vi "Get Unified Force.vi"(10 "diameter results":dbl[][](array[numeric]), 11 "force results":dbl[][](array[numeric])) -> (3 "unified force array":dbl[](array[numeric]))   [LabVIEW 2020]
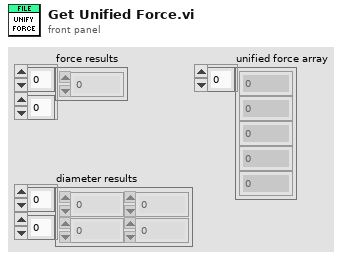
[diagram p1: front panel]
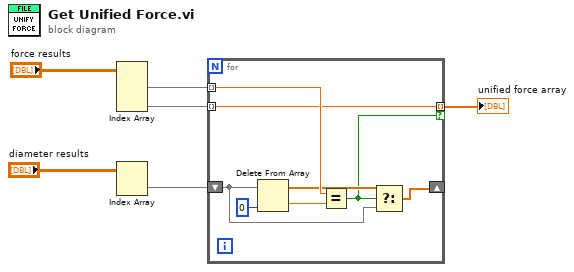
[diagram p0: block diagram]
diagram:
  n1 = Index Array(array="force results") -> (element #1=w2:dbl[], element #2=w3:dbl[])  [unwired: 4 in]
  n2 = Index Array(array="diameter results") -> (element=w4:dbl[])  [unwired: 2 in]
  n3 = for {
    tunnel: w2 -> [w14] mode=indexing
    tunnel: w3 -> [w13] mode=indexing
    tunnel: [w13] -> w6 mode=indexing if=w8
    shift-right: [w9] -> _
    shift-left: w4 -> [w10]
    n4 = Delete From Array(array=w10, index=0) -> (deleted portion=w12:dbl, array with subset deleted=w11:dbl[])  [unwired: 1 in]
    n5 = Equal?(x=w14, y=w12) -> (x = y?=w8:bool)
    n6 = Select(t=w11, s=w8, f=w10) -> (s? t:f=w9:dbl[])
  }
  "unified force array" <- w6
